vi "one_SPI_command.vi"() -> ()   [LabVIEW 2009]
panel:
  in  "chip delay":i32
  in  "Send continuous":bool
  in  "Send":bool
  in  "Id in":i32
  in  "Data":u32
  in  "register or channel":i32
  out "bucle":i32
  out "data read value":u32
  out "error out 2":errorcluster
  in  "error in (no error)":errorcluster
  out "hex integer string":string
  out "Id out":i32=72
  in  "Read physical":bool
  out "Data to send hex":string
  in  "Device":u16(ring) items=["Attenuation", "Clipping", "Enable channel", "Delay line", "ASIC"]
  in  "Read/#write":bool
  out "data out serial":string
  in  "stop":bool
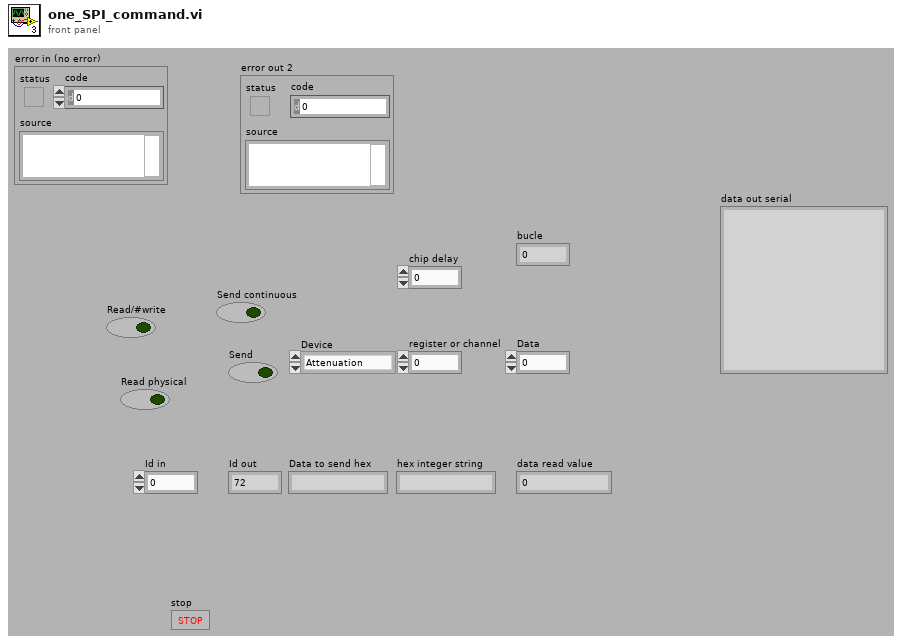
[diagram p1: front panel]
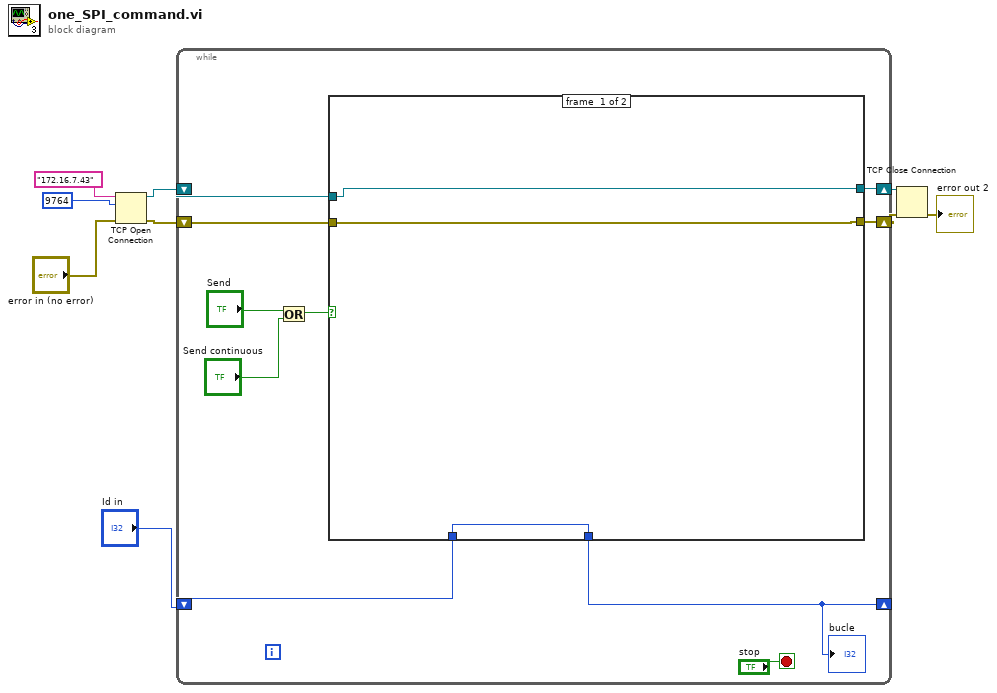
[diagram p0: block diagram]
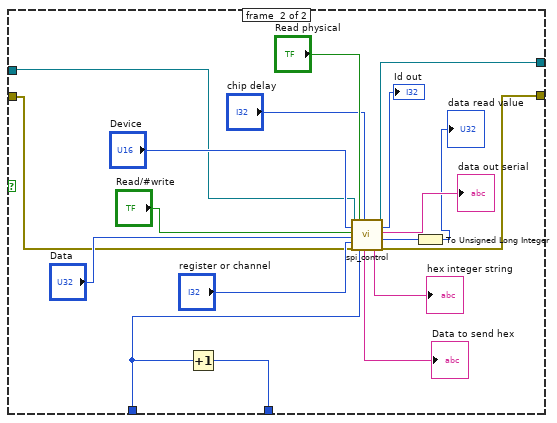
[diagram p2: hidden frame]
diagram:
  n1 = TCP Open Connection(address="172.16.7.43", remote port or service name=u16 9764, error in (no error)="error in (no error)") -> (connection ID=w5:refnum<k5>, error out=w4:errorcluster)  [unwired: 2 in]
  n2 = while {
    shift-right: [w19] -> w7
    shift-left: w4 -> [w17]
    shift-right: [w16] -> w6
    shift-left: w5 -> [w18]
    shift-right: [w13] -> _
    shift-left: "Id in" -> [w14]
    stop <- "stop" stop-if-true
    n3 = Or(x="Send", y="Send continuous") -> (x .or. y?=w12:bool)
    n4 = case shown="True" w12 {
      tunnel: [w21 w40] -> w19
      tunnel: w18 -> [w22 w26]
      tunnel: w17 -> [w21 w25]
      tunnel: [w22 w39] -> w16
      tunnel: w14 -> [w20 w24]
      tunnel: [w20 w28] -> w13
      frame #0 {
      }
      frame #1 {
        n5 = Increment(x=w24) -> (x+1=w28:i32)
        n6 = call "spi_control.vi"("connection ID"=w26, "Device"="Device", "Read/#write"="Read/#write", "Data"="Data", "Register or channel"="register or channel", "error out 3"=w25, "Read physical"="Read physical", "Id in"=w24, "chip delay"="chip delay") -> ("Data to send hex"=→"Data to send hex":string, "hex integer string"=→"hex integer string":string, "connection ID out"=w39:refnum<k5>, "Id out"=→"Id out":i32, "data out serial"=→"data out serial":string, "data read value"=w30:u32, "error out 2"=w40:errorcluster)  [unwired: 3 in, 1 out]
        n7 = To Unsigned Long Integer(number=w30) -> (unsigned 32bit integer=→"data read value":u32)
      }
    }
    "bucle" <- w13
  }
  n8 = TCP Close Connection(connection ID=w6, error in (no error)=w7) -> (error out=→"error out 2":errorcluster)  [unwired: 1 in, 1 out]
